vi "Post-Build Action.vi"(5 "Files Generated by Build":path[](array[path]), 6 "Top Level/Always Included VIs":path[](array[path]), 7 "Destination Path":path, 8 "error in (no error)":errorcluster, 9 "Target Name":string, 10 "Build Specification Name":string, 11 "Project Path":path) -> (0 "error out":errorcluster)   [LabVIEW 2014]
uses:
  <userlib>/_OpenG.lib/file/file.llb/Strip Path Extension - Path__ogtk.vi
  <userlib>/_OpenG.lib/file/file.llb/Convert File Extension (Path)__ogtk.vi
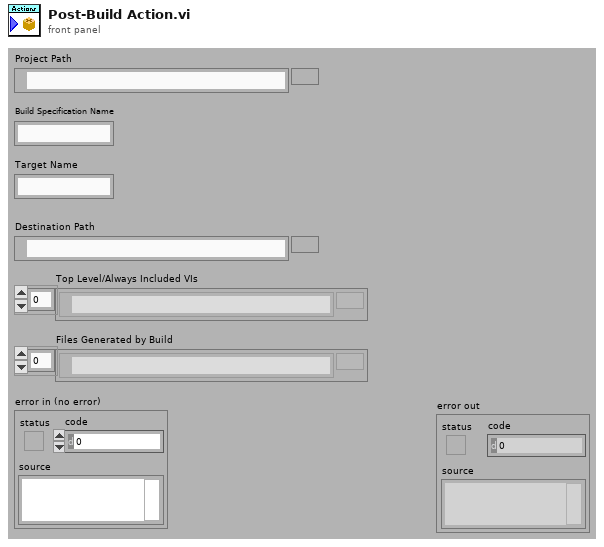
[diagram p1: front panel]
types:
  T1 = enum16{"CharacterArray", "FixedFileInfoCluster", "LanguageCode"}
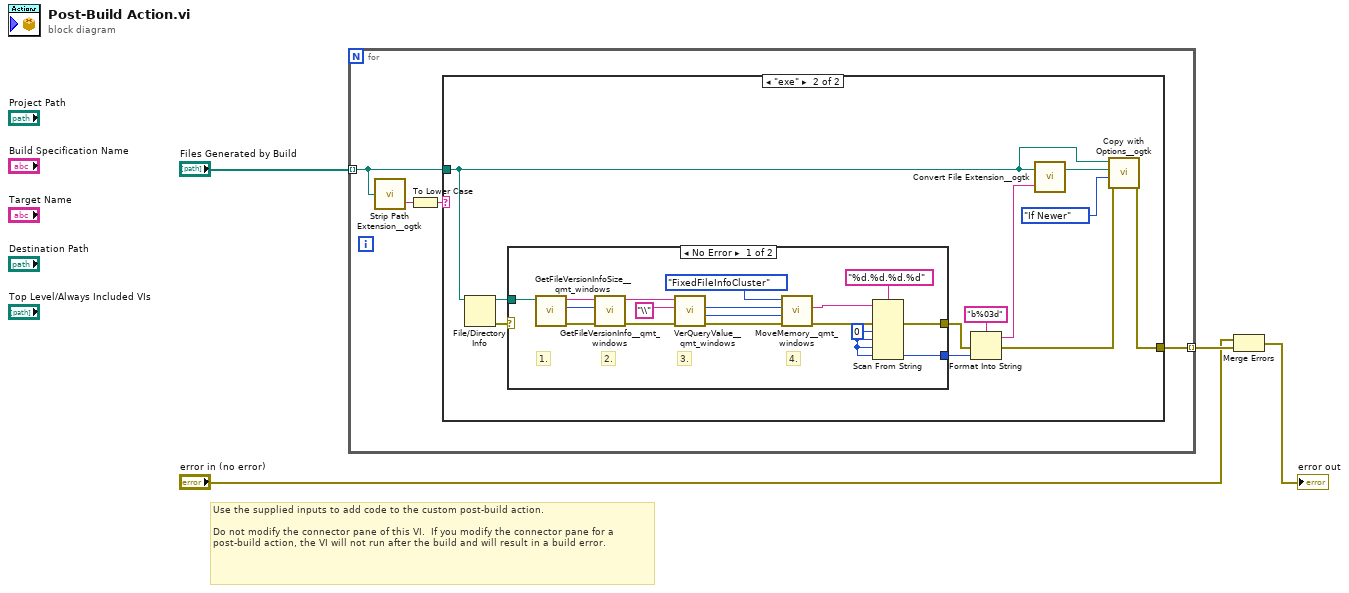
[diagram p0: block diagram]
diagram:
  # "Use the supplied inputs to add code to the custom post-build action.\n\nDo not modify the connector pane of this VI.  If you modify the connector pane for a post-build action, the VI will not run after the build and will result in a build error."
  n1 = for {
    tunnel: "Files Generated by Build" -> [w6] mode=indexing
    tunnel: [w5] -> w3 mode=indexing
    n2 = call-poly <userlib>:"Strip Path Extension__ogtk.vi"("path"=w6) -> ("extension"=w8:string)  [unwired: 1 out]
    n3 = To Lower Case(string=w8) -> (all lower case string=w7:string)
    n4 = case shown="\"exe\"" w7 {
      tunnel: w6 -> [_ w9]
      tunnel: [_ w10] -> w5
      frame Default {
      }
      frame "exe" {
        n5 = File/Directory Info(path=w9) -> (path out=w19:path, error out=w18:errorcluster)  [unwired: 1 in, 5 out]
        n6 = case shown="No Error" w18 {
          selector: w18 -> [_ w37]
          tunnel: w19 -> [w26 _]
          tunnel: [w21 w37] -> w16
          tunnel: [w20 _] -> w17
          frame No Error {
            w25 = 0 ("default value 1")
            # "4."
            # "3."
            # "2."
            # "1."
            n7 = call <userlib>:"GetFileVersionInfoSize__qmt_windows.vi"("Path"=w26) -> ("error out"=w29:errorcluster, "Size"=w28:i32, "lptstrFilename"=w30:string)  [unwired: 8 in]
            n8 = call <userlib>:"GetFileVersionInfo__qmt_windows.vi"("error in"=w29, "Size"=w28, "lptstrFilename"=w30) -> ("error out"=w31:errorcluster, "lpData"=w27:string)  [unwired: 7 in]
            n9 = call <userlib>:"VerQueryValue__qmt_windows.vi"("error in (no error)"=w31, "lpSubBlock"="\\", "lpData"=w27) -> ("error out"=w36:errorcluster, "puLen"=w33:i32, "lplpBuffer"=w34:i32)  [unwired: 6 in]
            n10 = call <userlib>:"MoveMemory__qmt_windows.vi"("error in (no error)"=w36, "puLen"=w33, "lplpBuffer"=w34, "Datatype"=T1."FixedFileInfoCluster") -> ("error out"=w23:errorcluster, "data"=w22:string)  [unwired: 6 in]
            n11 = Scan From String(format string="%d.%d.%d.%d", input string=w22, error in=w23, default 1=w25, default 2=w25, default 3=w25, default 4=w25) -> (error out=w21:errorcluster, output 4=w20:i32)  [unwired: 4 in, 2 out]
          }
          frame Error {
          }
        }
        n12 = Format Into String(format string="b%03d", error in=w16, w17) -> (resulting string=w15:string, error out=w11:errorcluster)  [unwired: 1 in]
        n13 = call-poly <userlib>:"Convert File Extension__ogtk.vi"("new ending (none)"=w15, "file name"=w9) -> ("new filename"=w13:path)  [unwired: 1 out]
        n14 = call <userlib>:"Copy with Options__ogtk.vi"("error in (no error)"=w11, "Replace Mode (Never)"=enum16{"Never", "Always", "If Newer"}."If Newer", "target path"=w13, "source path"=w9) -> ("error out"=w10:errorcluster)  [unwired: 6 in, 1 out]
      }
    }
  }
  n15 = Merge Errors("error in (no error)", w3) -> (→"error out":errorcluster)
